vi "Get Properties.vi"(10 "Pages":refnum<vi>[](array[refnum]), 11 "TabControl in":refnum<vi>) -> (1 "Array 2":string[](array[string]), 2 "Array":string[](array[string]), 3 "ControlsOnPage":refnum<vi>[](array[refnum]))   [LabVIEW 2013]
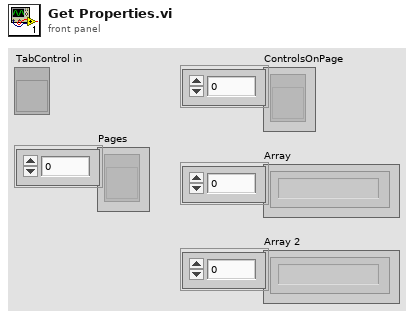
[diagram p1: front panel]
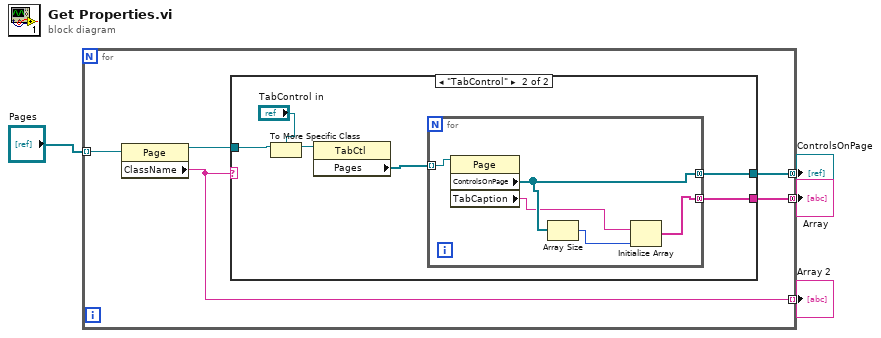
[diagram p0: block diagram]
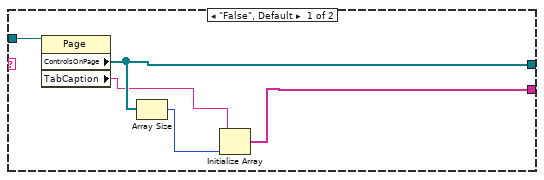
[diagram p2: hidden frame]
diagram:
  n1 = for {
    tunnel: "Pages" -> [w7] mode=indexing
    tunnel: [w9] -> w2 mode=concatenating
    tunnel: [w8] -> w3 mode=indexing
    tunnel: [w5] -> w4 mode=concatenating
    n2 = property class="Page"(reference=w7) -> (reference out=w6:refnum<vi>, "ClassName"=w8:string)  [unwired: 1 in, 1 out]
    n3 = case shown="\"TabControl\"" w8 {
      tunnel: [w13 w17] -> w9
      tunnel: w6 -> [w14 w20]
      tunnel: [w10 w16] -> w5
      frame "False", Default {
        n4 = property class="Page"(reference=w14) -> ("ControlsOnPage"=w13:refnum<vi>[], "TabCaption"=w11:string)  [unwired: 1 in, 2 out]
        n5 = Array Size(array=w13) -> (size(s)=w12:i32)
        n6 = Initialize Array(w11, w12) -> (w10:string[])
      }
      frame "TabControl" {
        n7 = To More Specific Class(target class="TabControl in", reference=w20) -> (specific class reference=w19:refnum<vi>)  [unwired: 1 in, 1 out]
        n8 = property class="TabCtl"(reference=w19) -> ("Pages"=w18:refnum<vi>[])  [unwired: 1 in, 2 out]
        n9 = for {
          tunnel: w18 -> [w25] mode=indexing
          tunnel: [w23] -> w17 mode=concatenating
          tunnel: [w21] -> w16 mode=concatenating
          n10 = property class="Page"(reference=w25) -> ("ControlsOnPage"=w23:refnum<vi>[], "TabCaption"=w22:string)  [unwired: 1 in, 2 out]
          n11 = Array Size(array=w23) -> (size(s)=w24:i32)
          n12 = Initialize Array(w22, w24) -> (w21:string[])
        }
      }
    }
  }
  "Array" <- w4
  "Array 2" <- w3
  "ControlsOnPage" <- w2
